vi "fake vi.vi"() -> ()   [LabVIEW 2016]
panel:
  in  "Tab Control":enum32{"Page 1", "Page 2"}(tab)
  in  "Boolean":bool
  in  "Numeric":dbl
  in  "Numeric 2":dbl
  in  "Boolean 2":bool
  in  "String":string
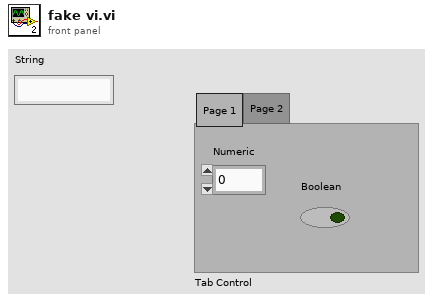
[diagram p1: front panel]
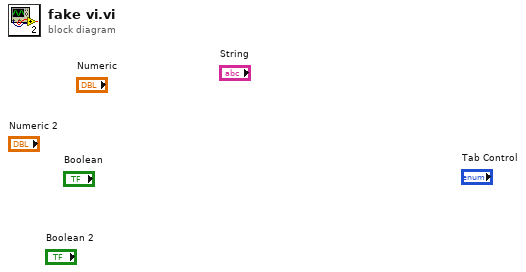
[diagram p0: block diagram]
diagram:
